vi "CheckForWHEREStrings.vi"(10 "Options":T1, 11 "ColumnNameEqualsValueFormat in":string) -> (3 "ColumnNameEqualsValueFormat out":string)   [LabVIEW 2020, in "ORM_DBC_Kdb.lvlib" / "DBC.lvclass"]
uses:
  DBC.lvclass
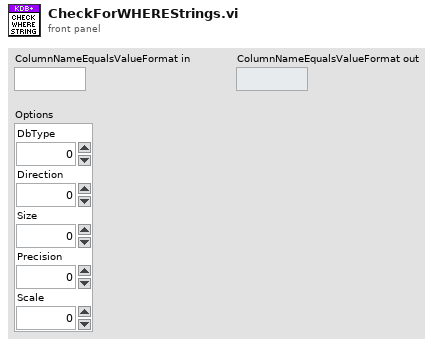
[diagram p1: front panel]
types:
  T1 = cluster{"DbType":i32, "Direction":i32, "Size":i32, "Precision":u8, "Scale":u8}
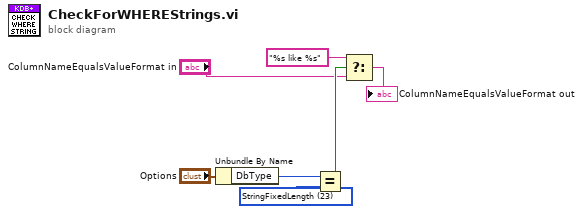
[diagram p0: block diagram]
diagram:
  w2 = 23 items=["AnsiString"=0, "Binary"=1, "Byte"=2, "Boolean"=3, "Currency"=4, "Date"=5, "DateTime"=6, "Decimal"=7, "Double"=8, "Guid"=9, "Int16"=10, "Int32"=11, "Int64"=12, "Object"=13, "SByte"=14, "Single"=15, "String"=16, "Time"=17, "UInt16"=18, "UInt32"=19, "UInt64"=20, "VarNumeric"=21, "AnsiStringFixedLength"=22, "StringFixedLength"=23, "Xml"=25, "DateTime2"=26, "DateTimeOffset"=27] ("DbType")
  n1 = Unbundle By Name("Options") -> ("DbType"=w3:i32)
  n2 = Equal?(x=w3, y=w2) -> (x = y?=w6:bool)
  n3 = Select(t="%s like %s", s=w6, f="ColumnNameEqualsValueFormat in") -> (s? t:f=→"ColumnNameEqualsValueFormat out":string)
